vi "Execute.vi"(8 "error in":errorcluster, 10 "Change Control Value CMD in":refnum<class "Change Control Value CMD.lvclass">, 11 "Object In":refnum<class>) -> (0 "error out":errorcluster, 3 "Object Out":refnum<class>)   [LabVIEW 2014, in "Humidifier Lib.lvlib" / "Change Control Value CMD.lvclass"]
doc: "Abstract method for accomplishing the execution of a command directed to an instrument object on the wire."
uses:
  Change Control Value CMD.lvclass
  Humidifier.lvclass
  Change Control Value CMD.lvclass/Change Control Value CMD.ctl
  Humidifier.lvclass/Humidifier.ctl
  Accessors/Write RH_.vi
  Accessors/Read Log Session.vi
  Accessors/Read ID.vi
  <userlib>/_Session Fwk/Session - Root.lvclass
  reusable/Session APIs/Session Log/System Log.lvclass
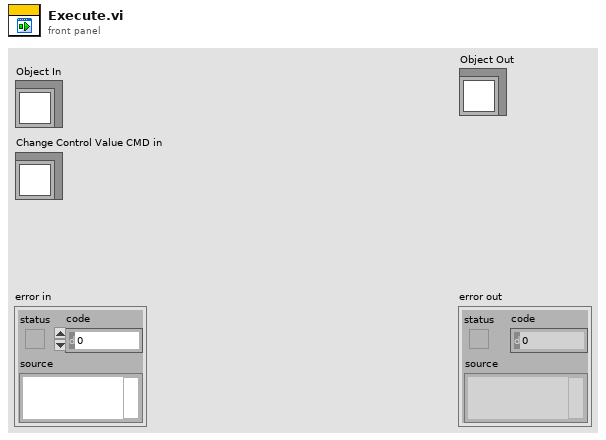
[diagram p1: front panel]
types:
  T1 = typedef "Session - Root.lvclass/Session Handle.ctl" = refnum<data-value>
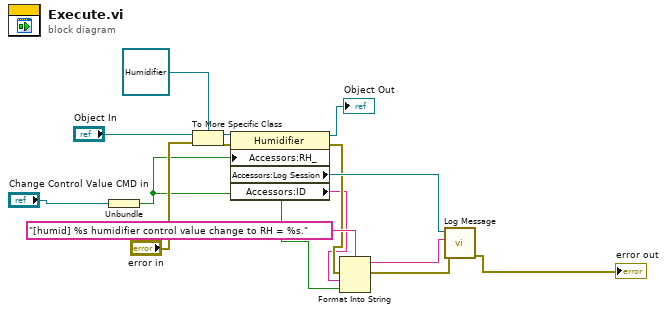
[diagram p0: block diagram]
diagram:
  n1 = Unbundle("Change Control Value CMD in") -> (w2:bool)
  n2 = To More Specific Class(target class=refnum<class "Humidifier.lvclass"> refnum ("Humidifier Lib.lvlib:Humidifier"), reference="Object In", error in="error in") -> (specific class reference=w13:refnum<class "Humidifier.lvclass">, error out=w12:errorcluster)
  n3 = property class="Humidifier"(reference=w13, error in=w12, "Accessors:RH_"=w2) -> (reference out=→"Object Out":refnum<class "Humidifier.lvclass">, error out=w4:errorcluster, "Accessors:Log Session"=w8:T1, "Accessors:ID"=w1:string)
  n4 = Format Into String(format string="[humid] %s humidifier control value change to RH = %s.", error in=w4, w1, w2) -> (resulting string=w6:string, error out=w5:errorcluster)  [unwired: 1 in]
  n5 = call "Log Message.vi"("error in"=w5, "MSG In"=w6, "session in"=w8) -> ("error out"=→"error out":errorcluster)  [unwired: 7 in, 1 out]
